vi "Set Custom Device Driver.vi"(8 "error in (no error)":errorcluster, 9 "Version":string="2020.0.0.0", 10 "Driver VIs":T1[](array[typedef]), 11 "BaseNodeType in":refnum<k39>) -> (0 "error out":errorcluster, 3 "BaseNodeType out":refnum<k39>)   [LabVIEW 2027, in "Embedded Data Logger System Explorer.lvlib"]
uses:
  Embedded Data Logger System Explorer.lvlib
  C:/NetCoreDLL/NationalInstruments.VeriStand.SystemStorage.dll
  NetCoreDLL/NationalInstruments.VeriStand.SystemStorage.dll
  <vilib>/NI VeriStand/Custom Device API/Path Type.ctl
  <vilib>/NI VeriStand/Custom Device API/Custom Device API.lvlib
  <vilib>/NI VeriStand/Custom Device API/Path Specification.ctl
  <vilib>/NI VeriStand/Custom Device API/Custom Device Supported Target.ctl
  <vilib>/NI VeriStand/Custom Device API/Custom Device Path Data.ctl
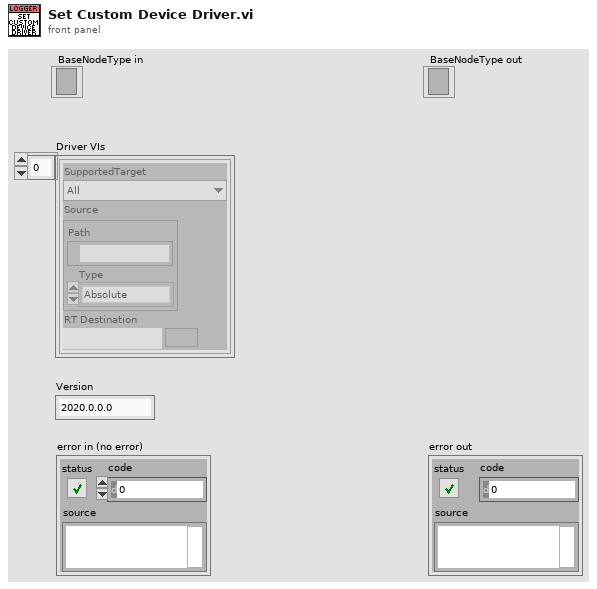
[diagram p1: front panel]
types:
  T1 = typedef "Custom Device API.lvlib/Custom Device Path Data.ctl" = cluster{"SupportedTarget":T2, "Source":T3, "RT Destination":path}
  T2 = typedef "Custom Device API.lvlib/Custom Device Supported Target.ctl" = enum16{"All", "PharLap", "VxWorks", "Windows", "Linux_32_ARM", "Linux_x64", "PharLap & Windows", "PharLap & VxWorks", "VxWorks & Windows"}
  T3 = typedef "Custom Device API.lvlib/Path Specification.ctl" = cluster{"Path":path, "Type":T4}
  T4 = typedef "Custom Device API.lvlib/Path Type.ctl" = enum16{"Absolute", "To Base", "To Common Data Dir", "To Application Data Dir"}
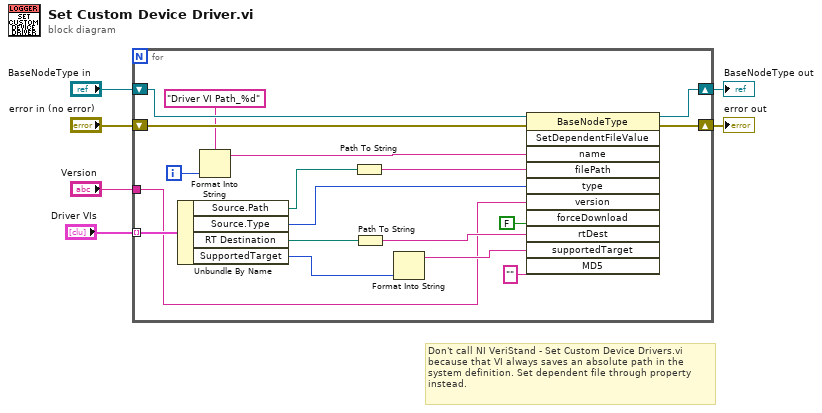
[diagram p0: block diagram]
diagram:
  # "Don't call NI VeriStand - Set Custom Device Drivers.vi\nbecause that VI always saves an absolute path in the\nsystem definition. Set dependent file through property\ninstead."
  n1 = for {
    shift-right: [w21] -> w4
    shift-left: "error in (no error)" -> [w24]
    shift-right: [w22] -> w3
    shift-left: "BaseNodeType in" -> [w23]
    tunnel: "Driver VIs" -> [w20] mode=indexing
    tunnel: "Version" -> [w7]
    i -> [w19]
    n2 = Unbundle By Name(w20) -> ("Source.Path"=w10:path, "Source.Type"=w17:T4, "RT Destination"=w9:path, "SupportedTarget"=w13:T2)
    n3 = Format Into String(format string="Driver VI Path_%d", w19) -> (resulting string=w18:string)  [unwired: 2 in, 1 out]
    n4 = Path To String(path=w10) -> (string=w11:string)
    n5 = Path To String(path=w9) -> (string=w8:string)
    n6 = Format Into String(w13) -> (resulting string=w12:string)  [unwired: 3 in, 1 out]
    n7 = invoke class="BaseNodeType" method="SetDependentFileValue"(reference=w23, error in=w24, "name"=w18, "filePath"=w11, "type"=w17, "version"=w7, "forceDownload"=FALSE, "rtDest"=w8, "supportedTarget"=w12, "MD5"="") -> (reference out=w22:refnum<k39>, error out=w21:errorcluster)  [unwired: 1 in, 9 out]
  }
  "error out" <- w4
  "BaseNodeType out" <- w3
